vi "23-2.vi"() -> ()   [LabVIEW 2019, in "23.lvlib"]
uses:
  23.lvlib
  Burrow/Burrow.lvclass
  Amphipod/Amphipod.lvclass
panel:
  out "Moves List":string[](array[string])
  in  "Sample?":bool
  in  "Sample Index":i32
  out "min energy":u64
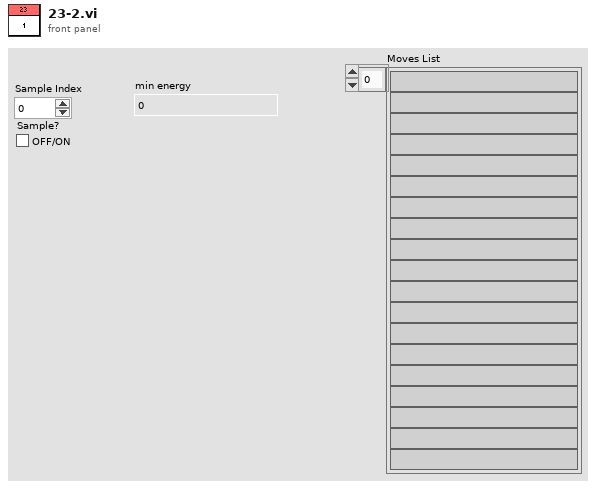
[diagram p1: front panel]
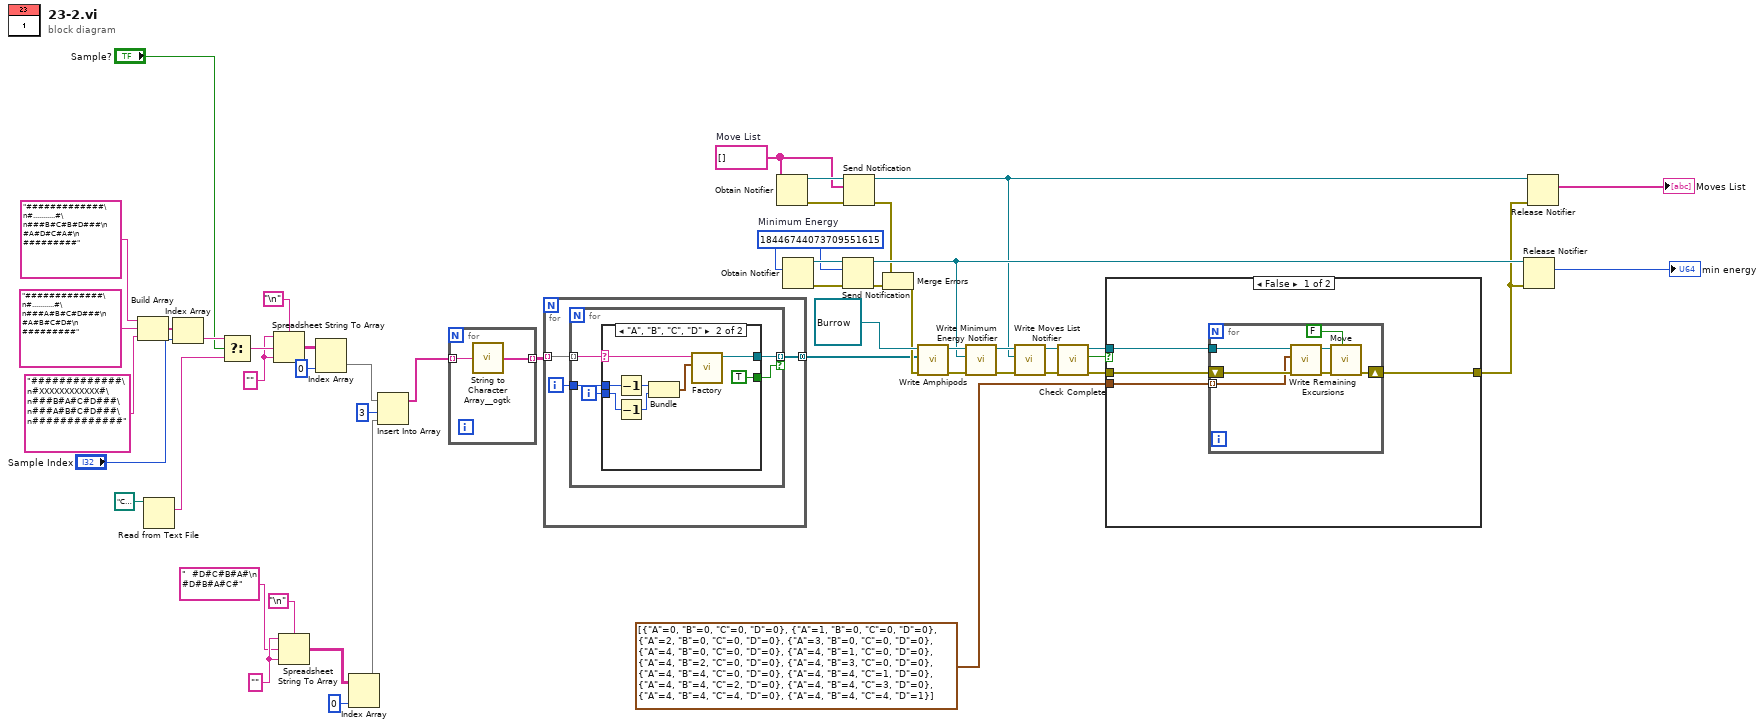
[diagram p0: block diagram]
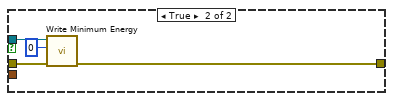
[diagram p3: hidden frame]
diagram:
  w9 = "" ("format string")
  w16 = "" ("format string")
  w28 = string[] []  # Move List
  w38 = u64 18446744073709551615  # Minimum Energy
  n1 = Build Array("#############\n#...........#\n###B#C#B#D###\n  #A#D#C#A#\n  #########", "#############\n#...........#\n###A#B#C#D###\n  #A#B#C#D#\n  #########", "#############\n#XXXXXXXXXXXX#\n###B#A#C#D###\n###A#B#C#D###\n#############") -> (w48:string[])
  n2 = Read from Text File(file (use dialog)=path "C:/Users/craig.walker/Documents/GitHub/lv2019-Advent-of-Code-2021/23/input.txt") -> (text=w43:string)  [unwired: 3 in, 3 out]
  n3 = Index Array(array=w48, index="Sample Index") -> (element=w44:string)
  n4 = Select(t=w44, s="Sample?", f=w43) -> (s? t:f=w17:string)
  n5 = Spreadsheet String To Array(delimiter (Tab)="\n", format string=w16, spreadsheet string=w17, array type (2D Dbl)=w16) -> (array=w14:string[][])
  n6 = Spreadsheet String To Array(delimiter (Tab)="\n", format string=w9, spreadsheet string="  #D#C#B#A#\n  #D#B#A#C#", array type (2D Dbl)=w9) -> (array=w5:string[][])
  n7 = Index Array(array=w14, index (col)=0 ("disabled index (col)")) -> (element=w4:string[])  [unwired: 1 in]
  n8 = Index Array(array=w5, index (col)=0 ("disabled index (col)")) -> (element=w3:string[])  [unwired: 1 in]
  n9 = Insert Into Array(array=w4, index=3, new element=w3) -> (w1:string[])
  n10 = for {
    tunnel: w1 -> [w52] mode=indexing
    tunnel: [w51] -> w13 mode=indexing
    n11 = call <userlib>:"String to Character Array__ogtk.vi"("Input String"=w52) -> ("Character Array"=w51:string[])
  }
  n12 = for {
    tunnel: w13 -> [w55] mode=indexing
    tunnel: [w53] -> w10 mode=concatenating
    i -> [w54]
    n13 = for {
      tunnel: w55 -> [w60] mode=indexing
      tunnel: w54 -> [w59]
      tunnel: [w57] -> w53 mode=indexing if=w56
      i -> [w58]
      n14 = case shown="\"A\", \"B\", \"C\", \"D\"" w60 {
        selector: w60 -> [_ w68]
        tunnel: w59 -> [_ w67]
        tunnel: w58 -> [_ w65]
        tunnel: [_ w63] -> w57
        tunnel: [_ TRUE] -> w56
        frame "False", Default {
        }
        frame "A", "B", "C", "D" {
          n15 = Decrement(x=w67) -> (x-1=w61:i32)
          n16 = Decrement(x=w65) -> (x-1=w64:i32)
          n17 = Bundle(w61, w64) -> (w66:cluster{i32, i32})  [unwired: 1 in]
          n18 = call "Factory.vi"("Position"=w66, "Type"=w68) -> ("Amphipod"=w63:refnum<class "Amphipod.lvclass">)  [unwired: 8 in, 1 out]
        }
      }
    }
  }
  n19 = Obtain Notifier(notification data type=w28) -> (notifier out=w29:refnum<notifier>, error out=w27:errorcluster)  [unwired: 3 in, 1 out]
  n20 = Obtain Notifier(notification data type=w38) -> (notifier out=w40:refnum<notifier>, error out=w39:errorcluster)  [unwired: 3 in, 1 out]
  n21 = Send Notification(notification=w38, notifier=w40, error in (no error)=w39) -> (notifier out=w34:refnum<notifier>, error out=w35:errorcluster)
  n22 = Send Notification(notification=w28, notifier=w29, error in (no error)=w27) -> (notifier out=w18:refnum<notifier>, error out=w23:errorcluster)
  n23 = Merge Errors(w23, w35) -> (w24:errorcluster)
  n24 = call-dynamic "Write Amphipods.vi"("error in (no error)"=w24, "Amphipods"=w10, "Burrow in"=refnum<class "Burrow.lvclass"> refnum) -> ("error out"=w37:errorcluster, "Burrow out"=w36:refnum<class "Burrow.lvclass">)  [unwired: 7 in]
  n25 = call-dynamic "Write Minimum Energy Notifier.vi"("error in (no error)"=w37, "Minimum Energy Notifier"=w34, "Burrow in"=w36) -> ("error out"=w20:errorcluster, "Burrow out"=w22:refnum<class "Burrow.lvclass">)  [unwired: 7 in]
  n26 = call-dynamic "Write Moves List Notifier.vi"("error in (no error)"=w20, "Moves List Notifier"=w18, "Burrow in"=w22) -> ("error out"=w19:errorcluster, "Burrow out"=w21:refnum<class "Burrow.lvclass">)  [unwired: 7 in]
  n27 = call-dynamic "Check Complete.vi"("error in (no error)"=w19, "Burrow in"=w21) -> ("error out"=w31:errorcluster, "Complete?"=w30:bool, "Burrow out"=w32:refnum<class "Burrow.lvclass">)  [unwired: 7 in]
  n28 = case shown="False" w30 {
    tunnel: [w72 w80] -> w25
    tunnel: w32 -> [w71 w83]
    tunnel: w31 -> [w70 w82]
    tunnel: cluster{"A":u8, "B":u8, "C":u8, "D":u8}[] [{"A"=0, "B"=0, "C"=0, "D"=0}, {"A"=1, "B"=0, "C"=0, "D"=0}, {"A"=2, "B"=0, "C"=0, "D"=0}, {"A"=3, "B"=0, "C"=0, "D"=0}, {"A"=4, "B"=0, "C"=0, "D"=0}, {"A"=4, "B"=1, "C"=0, "D"=0}, {"A"=4, "B"=2, "C"=0, "D"=0}, {"A"=4, "B"=3, "C"=0, "D"=0}, {"A"=4, "B"=4, "C"=0, "D"=0}, {"A"=4, "B"=4, "C"=1, "D"=0}, {"A"=4, "B"=4, "C"=2, "D"=0}, {"A"=4, "B"=4, "C"=3, "D"=0}, {"A"=4, "B"=4, "C"=4, "D"=0}, {"A"=4, "B"=4, "C"=4, "D"=1}] ("Remaining Excursions") -> [w69 _]
    frame False {
      n29 = for {
        tunnel: w71 -> [w75]
        shift-right: [w79] -> w72
        shift-left: w70 -> [w78]
        tunnel: w69 -> [w74] mode=indexing
        n30 = call-dynamic "Write Remaining Excursions.vi"("error in (no error)"=w78, "Remaining Excursions"=w74, "Burrow in"=w75) -> ("error out"=w77:errorcluster, "Burrow out"=w76:refnum<class "Burrow.lvclass">)  [unwired: 7 in]
        n31 = call-dynamic "Move.vi"("Part 1"=FALSE, "error in (no error)"=w77, "Burrow in"=w76) -> ("error out"=w79:errorcluster)  [unwired: 8 in]
      }
    }
    frame True {
      n32 = call-dynamic "Write Minimum Energy.vi"("error in (no error)"=w82, "Minimum Energy"=u64 0, "Burrow in"=w83) -> ("error out"=w80:errorcluster)  [unwired: 7 in, 1 out]
    }
  }
  n33 = Release Notifier(notifier=w34, error in (no error)=w25) -> (last notification=→"min energy":u64)  [unwired: 1 in, 2 out]
  n34 = Release Notifier(notifier=w18, error in (no error)=w25) -> (last notification=→"Moves List":string[])  [unwired: 1 in, 2 out]
